vi "Error 6003.vi"(8 "error in (no error)":errorcluster, 9 "rio status code":i32, 10 "register name":string) -> (0 "error out":errorcluster)   [LabVIEW 2020, in "FPGA Register IO.lvlib"]
uses:
  FPGA Register IO.lvlib
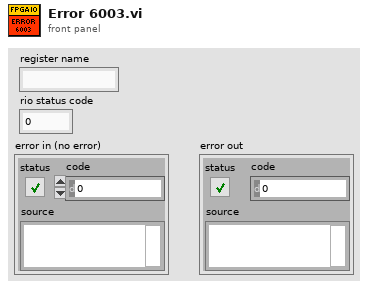
[diagram p1: front panel]
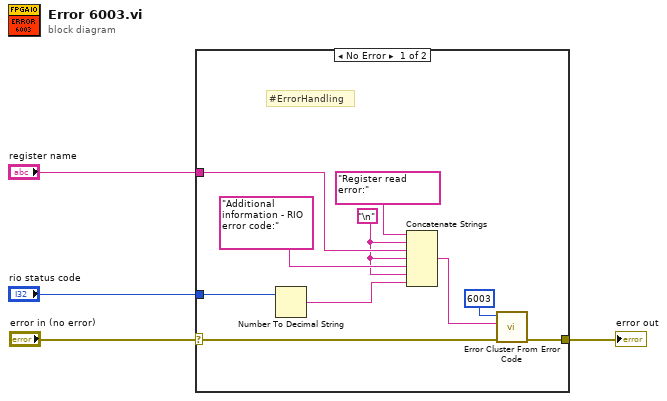
[diagram p0: block diagram]
diagram:
  n1 = case shown="No Error" "error in (no error)" {
    selector: "error in (no error)" -> [w11 w15]
    tunnel: [w12 w15] -> w4
    tunnel: "register name" -> [w9 _]
    tunnel: "rio status code" -> [w6 _]
    frame No Error {
      w7 = "\n"
      # "#ErrorHandling"
      n2 = Number To Decimal String(number=w6) -> (decimal integer string=w5:string)  [unwired: 1 in]
      n3 = Concatenate Strings("Register read error:" ("error message (\"\")"), w7, w9, w7, "Additional information - RIO error code:" ("string"), w7, w5) -> (w13:string)
      n4 = call <vilib>:"Error Cluster From Error Code.vi"("error in (no error)"=w11, "error message (\"\")"=w13, "error code (0)"=6003) -> ("error out"=w12:errorcluster)  [unwired: 6 in]
    }
    frame Error {
    }
  }
  "error out" <- w4
